vi "svx_Convert Waveform Graph Data to XY Graph Data.vi"(11 "Waveform Graph":cluster{"x0":dbl, "dx":dbl, "Y":dbl[]}[](array[cluster])) -> (3 "XY Graph":cluster{"X":dbl[], "Y":dbl[]}[](array[cluster]))   [LabVIEW 2017, in "SVX Waterfall Graph.xctl"]
uses:
  <vilib>/addons/_XControls/Waterfall Graph/SVX Waterfall Graph.xctl
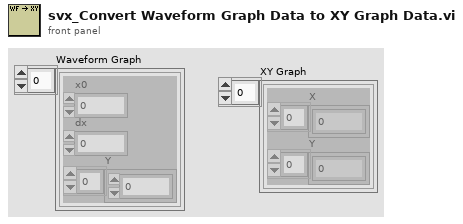
[diagram p1: front panel]
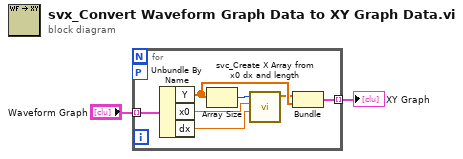
[diagram p0: block diagram]
diagram:
  n1 = for {
    tunnel: "Waveform Graph" -> [w9] mode=indexing
    tunnel: [w8] -> w1 mode=indexing
    workers-P: _ -> [_]
    n2 = Unbundle By Name(w9) -> ("Y"=w7:dbl[], "x0"=w5:dbl, "dx"=w3:dbl)
    n3 = Array Size(array=w7) -> (size(s)=w6:i32)
    n4 = call <vilib>:"svc_Create X Array from x0 dx and length.vi"("dx"=w3, "x0"=w5, "length"=w6) -> ("X"=w4:dbl[])  [unwired: 8 in]
    n5 = Bundle("X"=w4, "Y"=w7) -> (w8:cluster{"X":dbl[], "Y":dbl[]})  [unwired: 1 in]
  }
  "XY Graph" <- w1
